vi "GetConfig.vi"(8 "error in (no error)":errorcluster, 11 "Controlador in":refnum<class "Controlador.lvclass">) -> (0 "error out":errorcluster, 2 "String":string, 3 "Controlador out":refnum<class "Controlador.lvclass">)   [LabVIEW 2018, in "Controlador.lvclass"]
uses:
  Controlador.lvclass
  Controlador.lvclass/Controlador.ctl
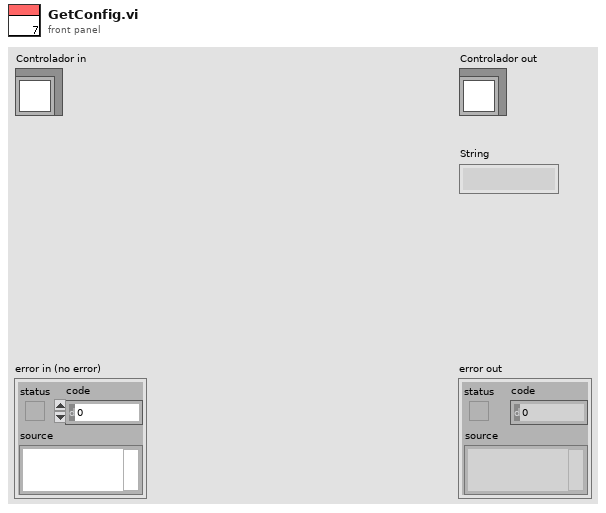
[diagram p1: front panel]
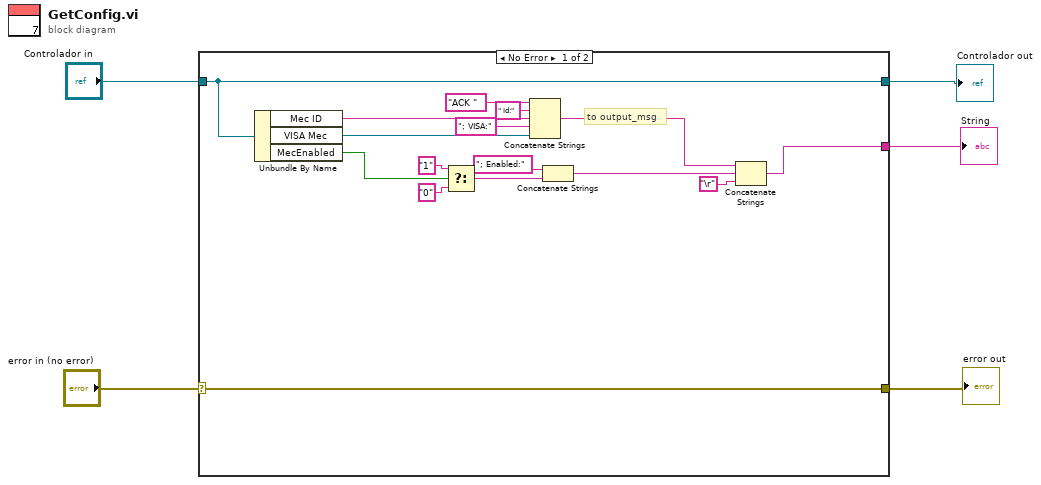
[diagram p0: block diagram]
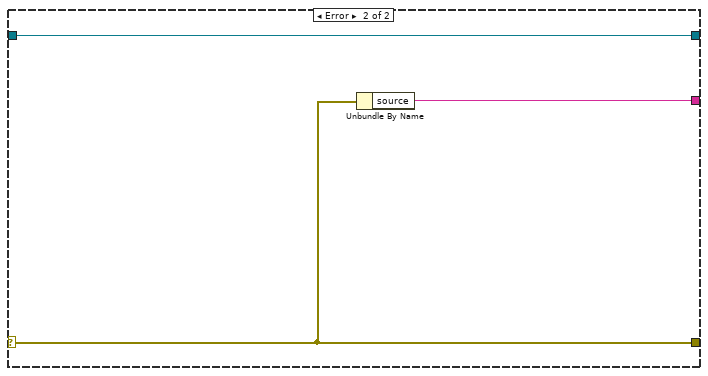
[diagram p2: hidden frame]
diagram:
  n1 = case shown="No Error" "error in (no error)" {
    selector: "error in (no error)" -> [w16 w24]
    tunnel: [w16 w24] -> w3
    tunnel: [w17 w23] -> w5
    tunnel: "Controlador in" -> [w6 w22]
    tunnel: [w6 w22] -> w1
    frame No Error {
      # "to output_msg"
      n2 = Unbundle By Name(w6) -> ("Mec ID"=w8:string, "VISA Mec"=w9:refnum<visa-resource-name>, "MecEnabled"=w7:bool)
      n3 = Select(t="1", s=w7, f="0") -> (s? t:f=w12:string)
      n4 = Concatenate Strings("ACK " ("string"), " Id:" ("string"), w8, "; VISA:" ("string"), w9) -> (w18:string)
      n5 = Concatenate Strings("; Enabled:" ("string"), w12) -> (w11:string)
      n6 = Concatenate Strings(w18, w11, "\r") -> (w17:string)
    }
    frame Error {
      n7 = Unbundle By Name(w24) -> ("source"=w23:string)
    }
  }
  "error out" <- w3
  "Controlador out" <- w1
  "String" <- w5
